vi "Gantry Class Sandbox.vi"() -> ()   [LabVIEW 2011]
uses:
  Gantry Class.lvclass
  Vec3d Class/Vec3d Class.lvclass
panel:
  in  "Config Folder":path=path "C:/Users/Husker/Desktop/gantry/Config"
  out "error out":errorcluster
  # "This VI tests the gantry class"
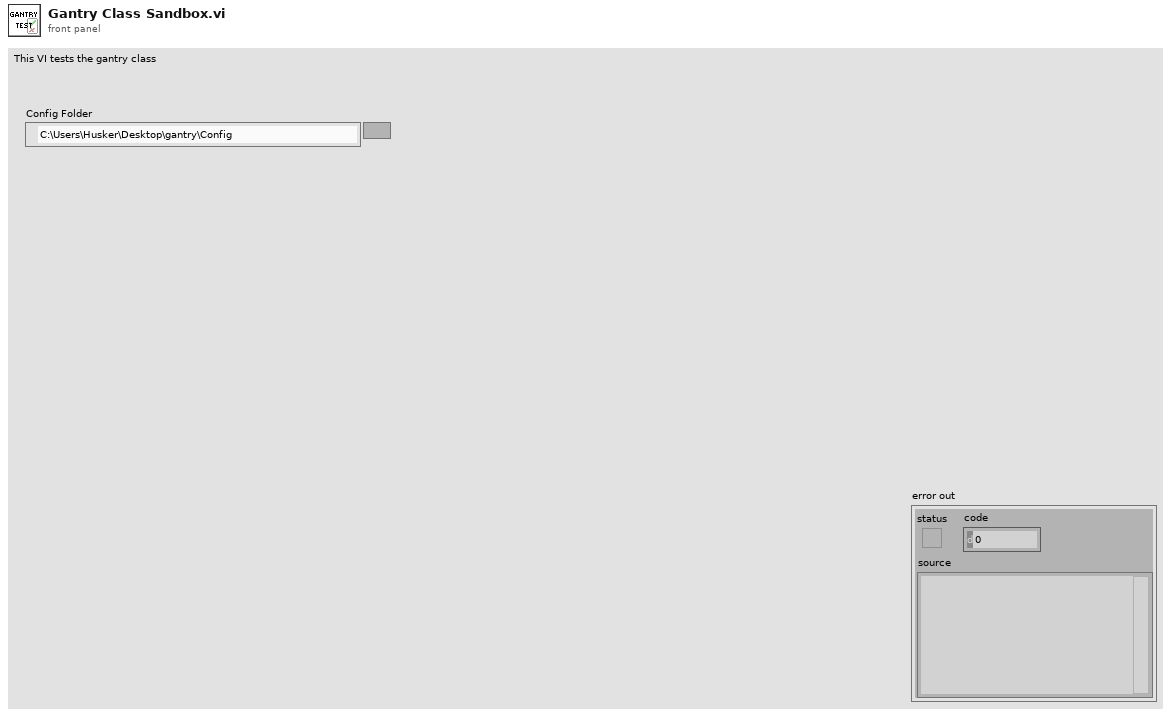
[diagram p1: front panel]
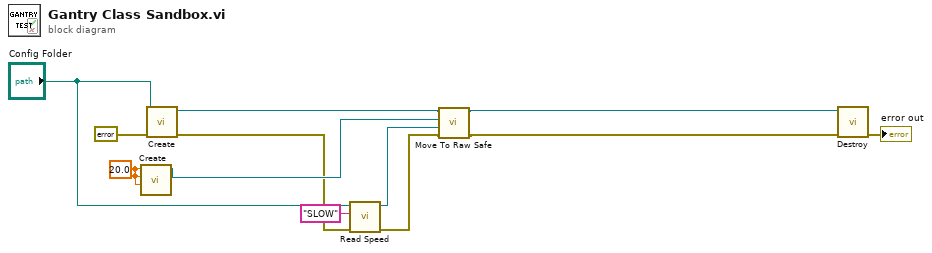
[diagram p0: block diagram]
diagram:
  w7 = 20.0 ("X")
  n1 = call "Create.vi"("Z"=w7, "Y"=w7, "X"=w7) -> ("Vec3d Class out"=w6:refnum<class "Vec3d Class.lvclass">)  [unwired: 7 in, 1 out]
  n2 = call "Create.vi"("error in (no error)"=errorcluster {"status"=FALSE, "code"=0, "source"=""} ("error constant"), "Config Folder"="Config Folder") -> ("error out"=w4:errorcluster, "Gantry Class out"=w10:refnum<class "Gantry Class.lvclass">)  [unwired: 8 in]
  n3 = call "Read Speed.vi"("error in (no error)"=w4, "Speeds Label"="SLOW", "Config Files Path"="Config Folder") -> ("error out"=w3:errorcluster, "Vec3d out"=w5:refnum<class "Vec3d Class.lvclass">)  [unwired: 7 in]
  n4 = call "Move To Raw Safe.vi"("error in (no error)"=w3, "Speed"=w5, "Position"=w6, "Gantry Class in"=w10) -> ("error out"=w8:errorcluster, "Gantry Class out"=w9:refnum<class "Gantry Class.lvclass">)  [unwired: 6 in]
  n5 = call "Destroy.vi"("error in (no error)"=w8, "Gantry Class in"=w9) -> ("error out"=→"error out":errorcluster)  [unwired: 9 in]
